vi "Create Tree.vi"(7 "Parent ID (empty)":string, 8 "Error In":errorcluster, 10 "Name":string, 11 "Tree Manager":refnum<data-value>) -> (0 "Error Out":errorcluster, 3 "Tree Manager":refnum<data-value>, 5 "Unique ID":string)   [LabVIEW 2017, in "Tree API.lvlib" / "Tree.lvclass"]
doc: "Create a new Tree in the Tree Manager and assign to it a Unique ID. Use this Unique ID to interact with this tree.\n\nYou can provide the optional Parent ID input if you want to create the Child Tree directly under already existing Parent.\n\n<b>WARNING</b> The name Attr is reserved by the Tree API. Do not use that name for your Trees. Flattening to XML requires the Tree Names to contain no white spaces. All white spaces will be replaced with underscore characters when flattening."
uses:
  Tree.lvclass
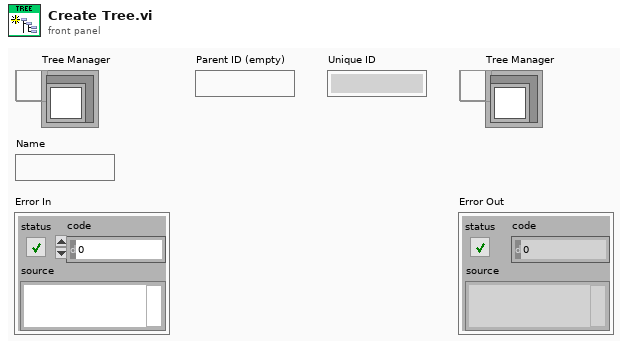
[diagram p1: front panel]
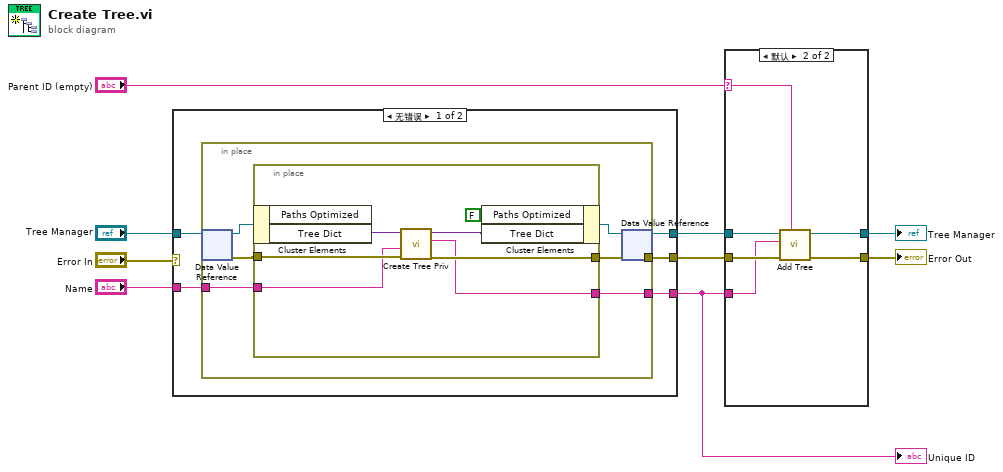
[diagram p0: block diagram]
diagram:
  n1 = case shown="无错误" "Error In" {
    selector: "Error In" -> [_ w28]
    tunnel: "Tree Manager" -> [w14 w29]
    tunnel: [w13 w29] -> w7
    tunnel: [w12 w28] -> w8
    tunnel: "Name" -> [w11 _]
    tunnel: [w10 _] -> w5
    frame No Error {
      n2 = in-place {
        in-place-border: [w19] -> w12
        in-place-border: w11 -> [w17]
        in-place-border: [w16] -> w10
        n3 = in-place-dvr #1(w14) -> (w20:refnum<class "Tree.lvclass">, w15:errorcluster)
        n4 = in-place {
          in-place-border: [w24] -> w19
          in-place-border: w15 -> [w25]
          in-place-border: w17 -> [w22]
          in-place-border: [w23] -> w16
          n5 = in-place-cluster #2(w20) -> ("Tree Dict"=w27:variant)  [unwired: 1 out]
          n6 = call "Create Tree Priv.vi"("Error In"=w25, "Name"=w22, "Tree Dictionary In"=w27) -> ("Error Out"=w24:errorcluster, "Unique ID"=w23:string, "Tree Dictionary Out"=w26:variant)  [unwired: 6 in]
          n7 = in-place-cluster #2("Paths Optimized"=FALSE, "Tree Dict"=w26) -> (w18:refnum<class "Tree.lvclass">)
        }
        n8 = in-place-dvr #1(w18) -> (w13:refnum<data-value>)  [unwired: 1 out]
      }
    }
    frame Error {
    }
  }
  "Unique ID" <- w5
  n9 = case shown="默认" "Parent ID (empty)" {
    selector: "Parent ID (empty)" -> [_ w33]
    tunnel: w8 -> [w30 w37]
    tunnel: [w30 w36] -> w1
    tunnel: w7 -> [w31 w35]
    tunnel: [w31 w34] -> w2
    tunnel: w5 -> [_ w32]
    frame "" {
    }
    frame Default {
      n10 = call "Add Tree.vi"("Parent ID"=w33, "Error In"=w37, "Child ID"=w32, "Tree Manager"=w35) -> ("Error Out"=w36:errorcluster, "Tree Manager"=w34:refnum<data-value>)  [unwired: 6 in]
    }
  }
  "Tree Manager" <- w2
  "Error Out" <- w1
